vi "mediaplaer-test_ver.vi"() -> ()   [LabVIEW 2010]
panel:
  in  "schließe":bool
  in  "Pfad":path
  out "SAMIStyle":string
  out "ende?":bool
  in  "schließen":bool
  in  "stop":bool
  in  "pause":bool
  in  "play":bool
  in  "Schieberegler":dbl(slide) scale=0.0..100.0
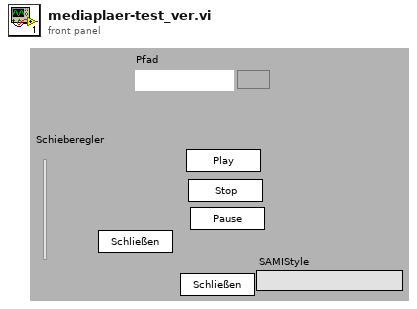
[diagram p1: front panel]
types:
  T1 = enum32{"play", "stop", "pause", "lautstärke veränderung"}
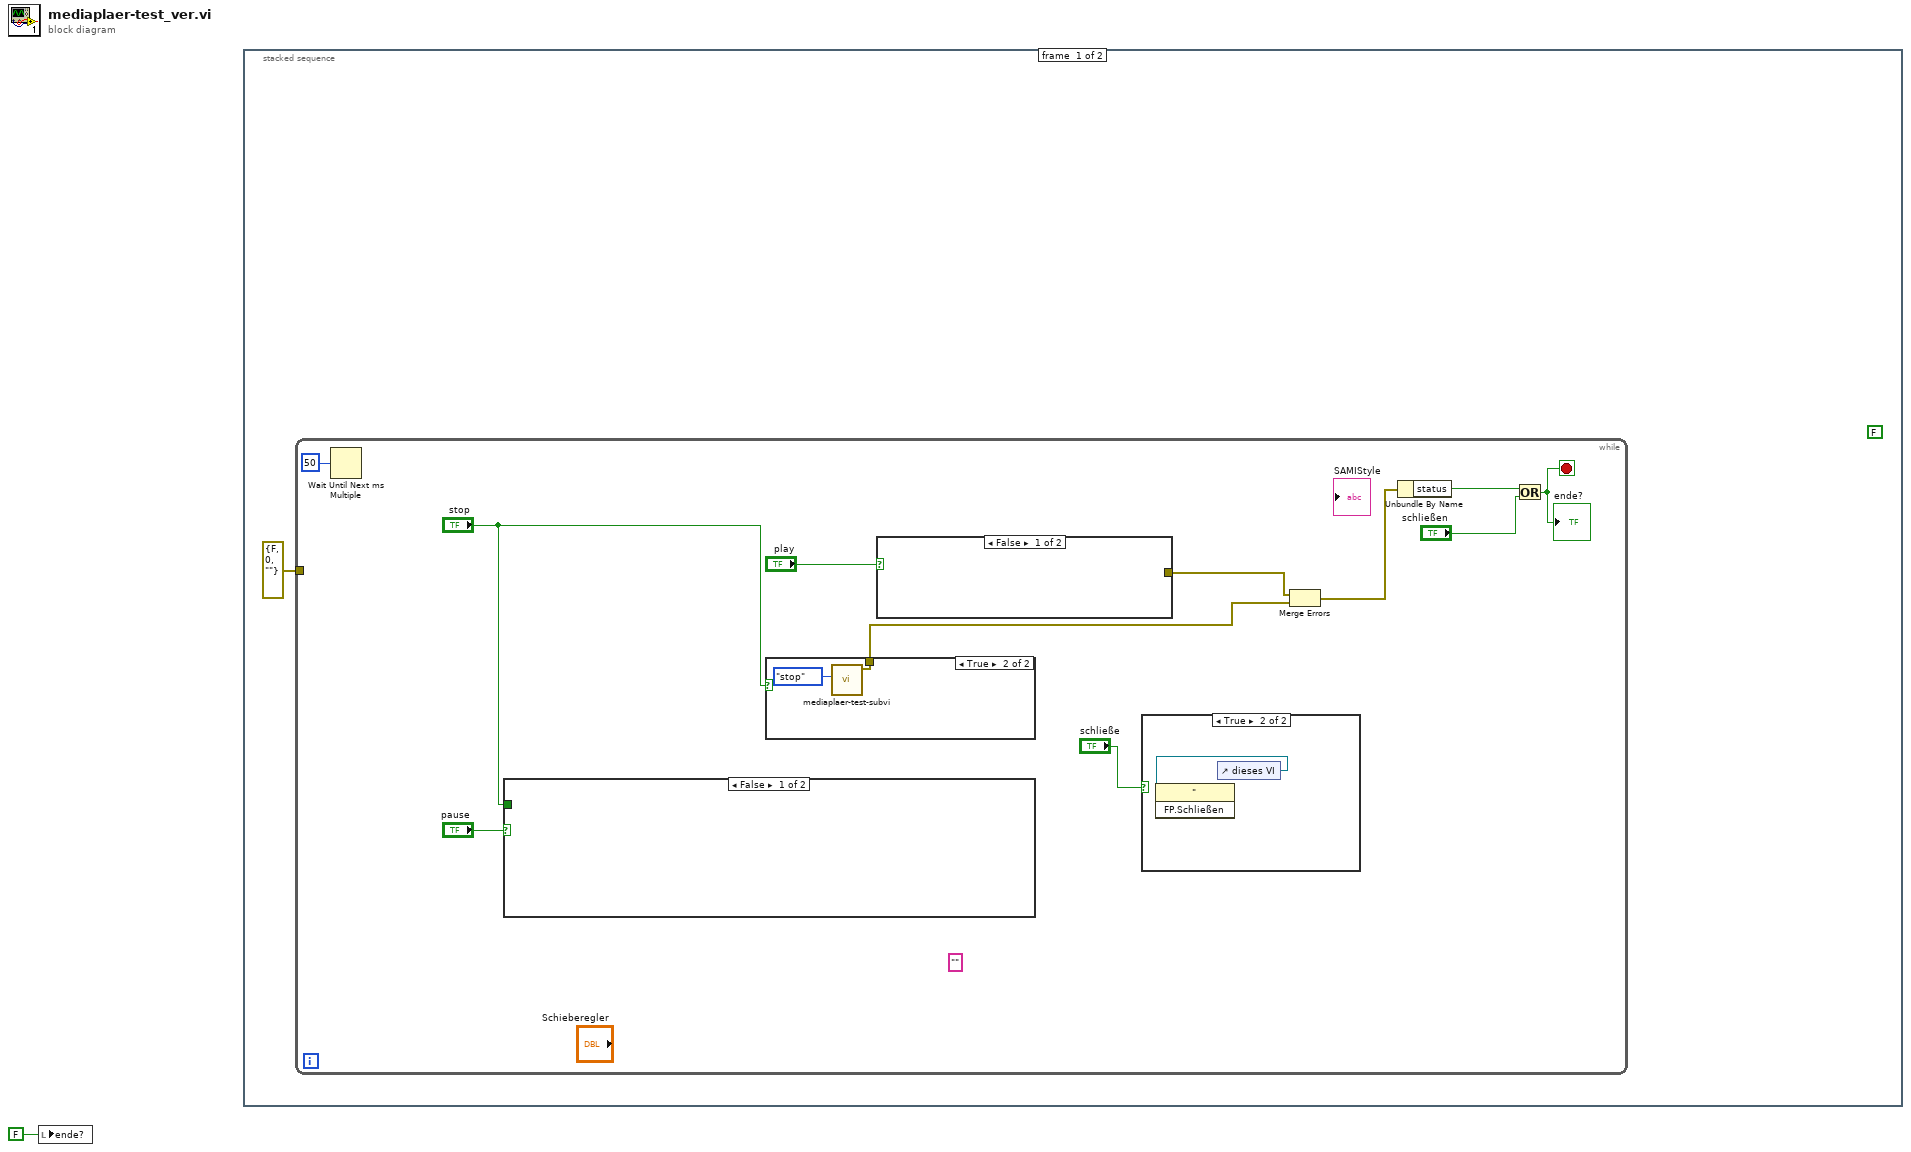
[diagram p0: block diagram]
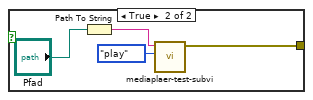
[diagram p5: hidden frame]
diagram:
  n1 = local write "ende?"(FALSE ("ende?")) -> ()
  n2 = stacked-sequence {
    frame #0 {
      (unwired) FALSE ("Neue Instanz öffnen (False)")
      n3 = while {
        tunnel: errorcluster {"status"=FALSE, "code"=0, "source"=""} ("error out") -> [_]
        stop <- w7 stop-if-true
        (unwired) "" ("uiMode")
        n4 = Wait Until Next ms Multiple(millisecond multiple=u32 50 ("Vielfache von ms")) -> ()  [unwired: 1 out]
        n5 = case shown="FALSE" "pause" {
          tunnel: "stop" -> [_ _]
          frame False {
          }
          frame True {
          }
        }
        n6 = case shown="TRUE" "stop" {
          tunnel: [_ w15] -> w5
          frame False {
          }
          frame True {
            n7 = call "mediaplaer-test-subvi.vi"("Optionsfelder"=T1."stop") -> ("Fehler (Ausgang)"=w15:errorcluster)  [unwired: 10 out]
          }
        }
        n8 = case shown="FALSE" "play" {
          tunnel: [_ w18] -> w6
          frame False {
          }
          frame True {
            n9 = Path To String(path="Pfad") -> (string=w19:string)
            n10 = call "mediaplaer-test-subvi.vi"("Optionsfelder"=T1."play", "url"=w19) -> ("Fehler (Ausgang)"=w18:errorcluster)  [unwired: 1 in, 8 out]
          }
        }
        n11 = case shown="TRUE" "schließe" {
          frame False {
          }
          frame True {
            n12 = control-ref of="dieses VI"() -> (w14:refnum<vi>)
            n13 = invoke class="\"" method="FP.Schließen"(reference=w14) -> ()  [unwired: 2 in, 3 out]
          }
        }
        n14 = Merge Errors(w6, w5) -> (w4:errorcluster)
        n15 = Unbundle By Name(w4) -> ("status"=w8:bool)
        n16 = Or(x=w8, y="schließen") -> (x .or. y?=w7:bool)
        "ende?" <- w7
      }
    }
    frame #1 {
    }
  }
